vi "Process Data PID 1 control.vi"(0 "Target Pos Set":i32, 1 "A_Pos":i32, 2 "Target Velo Set":i32, 3 "A_Vel":i32, 4 "Force_mode_L":bool, 5 "dt IN (s)":dbl=-1.0 format="%.8f", 7 "Actual_Cur_1":i16) -> (14 "Targer Cur L":i16 caption="Target Cur L", 19 "dt OUT (s)":dbl format="%.8f")   [LabVIEW 2019]
uses:
  <vilib>/addons/control/pid/pid.llb/PID (DBL).vi
  <vilib>/addons/control/pid/NI_PID_pid.lvlib
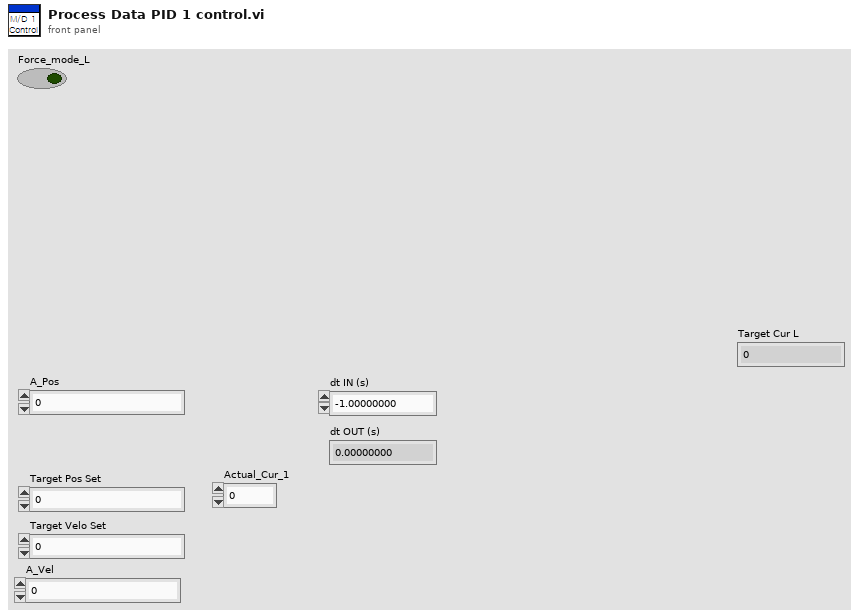
[diagram p1: front panel]
types:
  T1 = cluster{"proportional gain (Kc)":dbl, "integral time (Ti, min)":dbl, "derivative time (Td, min)":dbl}
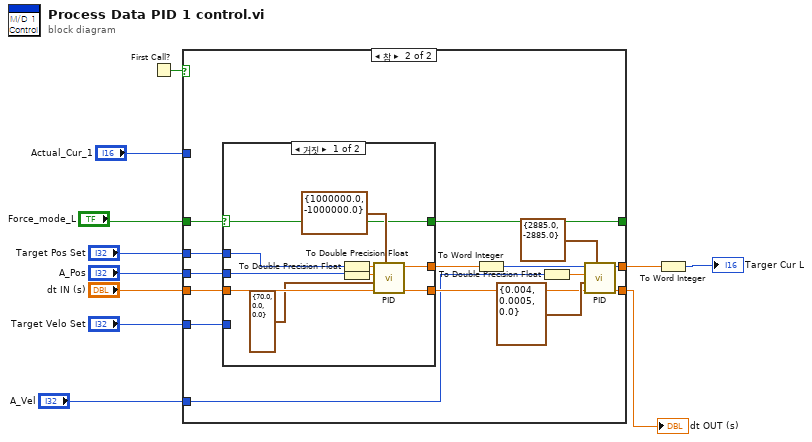
[diagram p0: block diagram]
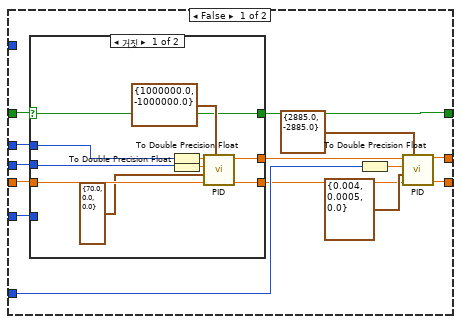
[diagram p2: hidden frame]
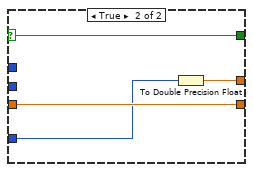
[diagram p3: hidden frame]
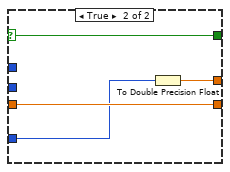
[diagram p4: hidden frame]
diagram:
  n1 = First Call?() -> (First Call?: T/F=w5:bool)
  n2 = case shown="참" w5 {
    tunnel: [w20 w54] -> w4
    tunnel: "Target Pos Set" -> [w22 w53]
    tunnel: "dt IN (s)" -> [w24 w52]
    tunnel: "A_Pos" -> [w23 w51]
    tunnel: "Target Velo Set" -> [w25 w50]
    tunnel: "Force_mode_L" -> [w18 w49]
    tunnel: [w21 w48] -> w3
    tunnel: [w19 w41] -> _
    tunnel: "Actual_Cur_1" -> [_ _]
    tunnel: "A_Vel" -> [w17 w40]
    frame False {
      n3 = case shown="거짓" w18 {
        selector: w18 -> [w27 w36]
        tunnel: [w35 w37] -> w14
        tunnel: [w34 w39] -> w12
        tunnel: w22 -> [w30 _]
        tunnel: w24 -> [w33 w39]
        tunnel: w25 -> [_ w38]
        tunnel: [w27 w36] -> w19
        tunnel: w23 -> [w26 _]
        frame False {
          n4 = To Double Precision Float(number=w30) -> (double precision float=w32:dbl)
          n5 = To Double Precision Float(number=w26) -> (double precision float=w31:dbl)
          n6 = call-poly <vilib>:"PID.vi"("output range"=cluster{"output high":dbl, "output low":dbl} {"output high"=1000000.0, "output low"=-1000000.0} ("output range 2"), "dt (s)"=w33, "PID gains"=T1 {"proportional gain (Kc)"=70.0, "integral time (Ti, min)"=0.0, "derivative time (Td, min)"=0.0} ("PID gains 2"), "process variable"=w31, "setpoint"=w32) -> ("dt out (s)"=w34:dbl, "output"=w35:dbl)  [unwired: 5 in]
        }
        frame True {
          n7 = To Double Precision Float(number=w38) -> (double precision float=w37:dbl)
        }
      }
      n8 = To Double Precision Float(number=w17) -> (double precision float=w15:dbl)
      n9 = call-poly <vilib>:"PID.vi"("output range"=cluster{"output high":dbl, "output low":dbl} {"output high"=2885.0, "output low"=-2885.0}, "dt (s)"=w12, "PID gains"=T1 {"proportional gain (Kc)"=0.004, "integral time (Ti, min)"=0.0005, "derivative time (Td, min)"=0.0}, "process variable"=w15, "setpoint"=w14) -> ("dt out (s)"=w20:dbl, "output"=w21:dbl)  [unwired: 5 in]
    }
    frame True {
      n10 = case shown="거짓" w49 {
        selector: w49 -> [w55 w65]
        tunnel: [w64 w66] -> w45
        tunnel: [w63 w68] -> w43
        tunnel: w53 -> [w58 _]
        tunnel: w52 -> [w62 w68]
        tunnel: w51 -> [w59 _]
        tunnel: w50 -> [_ w67]
        tunnel: [w55 w65] -> w41
        frame False {
          n11 = To Double Precision Float(number=w58) -> (double precision float=w61:dbl)
          n12 = To Double Precision Float(number=w59) -> (double precision float=w60:dbl)
          n13 = call-poly <vilib>:"PID.vi"("output range"=cluster{"output high":dbl, "output low":dbl} {"output high"=1000000.0, "output low"=-1000000.0} ("output range 2"), "dt (s)"=w62, "PID gains"=T1 {"proportional gain (Kc)"=70.0, "integral time (Ti, min)"=0.0, "derivative time (Td, min)"=0.0} ("PID gains 2"), "process variable"=w60, "setpoint"=w61) -> ("dt out (s)"=w63:dbl, "output"=w64:dbl)  [unwired: 5 in]
        }
        frame True {
          n14 = To Double Precision Float(number=w67) -> (double precision float=w66:dbl)
        }
      }
      n15 = To Double Precision Float(number=w40) -> (double precision float=w46:dbl)
      n16 = call-poly <vilib>:"PID.vi"("output range"=cluster{"output high":dbl, "output low":dbl} {"output high"=2885.0, "output low"=-2885.0}, "dt (s)"=w43, "PID gains"=T1 {"proportional gain (Kc)"=0.004, "integral time (Ti, min)"=0.0005, "derivative time (Td, min)"=0.0}, "process variable"=w46, "setpoint"=w45) -> ("dt out (s)"=w54:dbl, "output"=w42:dbl)  [unwired: 5 in]
      n17 = To Word Integer(number=w42) -> (16bit integer=w48:i16)
    }
  }
  "dt OUT (s)" <- w4
  n18 = To Word Integer(number=w3) -> (16bit integer=→"Targer Cur L":i16)
